vi "Graphs.vi"() -> ()   [LabVIEW 2020, in "Database Lib.lvlib"]
uses:
  Database Lib.lvlib
  <vilib>/Analysis/baseanly.llb/Mean (DBL).vi
  <vilib>/Analysis/NI_AALBase.lvlib
panel:
  out "XY Graph":cluster{"X":dbl, "Y":dbl}[](graph)
  out "Tab Control":enum32{"Histogram", "Length-Width", "Grading"}(tab)
  out "Diameter Histogram":cluster{"subarray":dbl[], dbl[]}(graph)
  in  "Menu":enum32{"Histogram", "Length-Width", "Grading"}(radio)
  in  "Close":bool
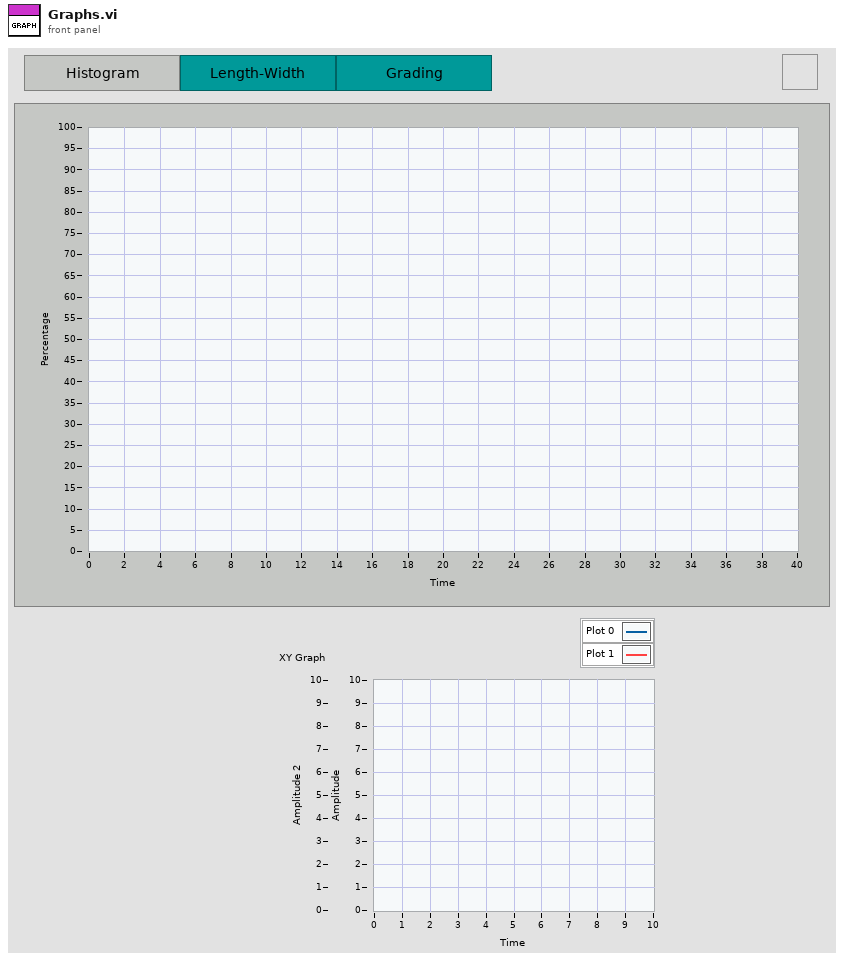
[diagram p1: front panel]
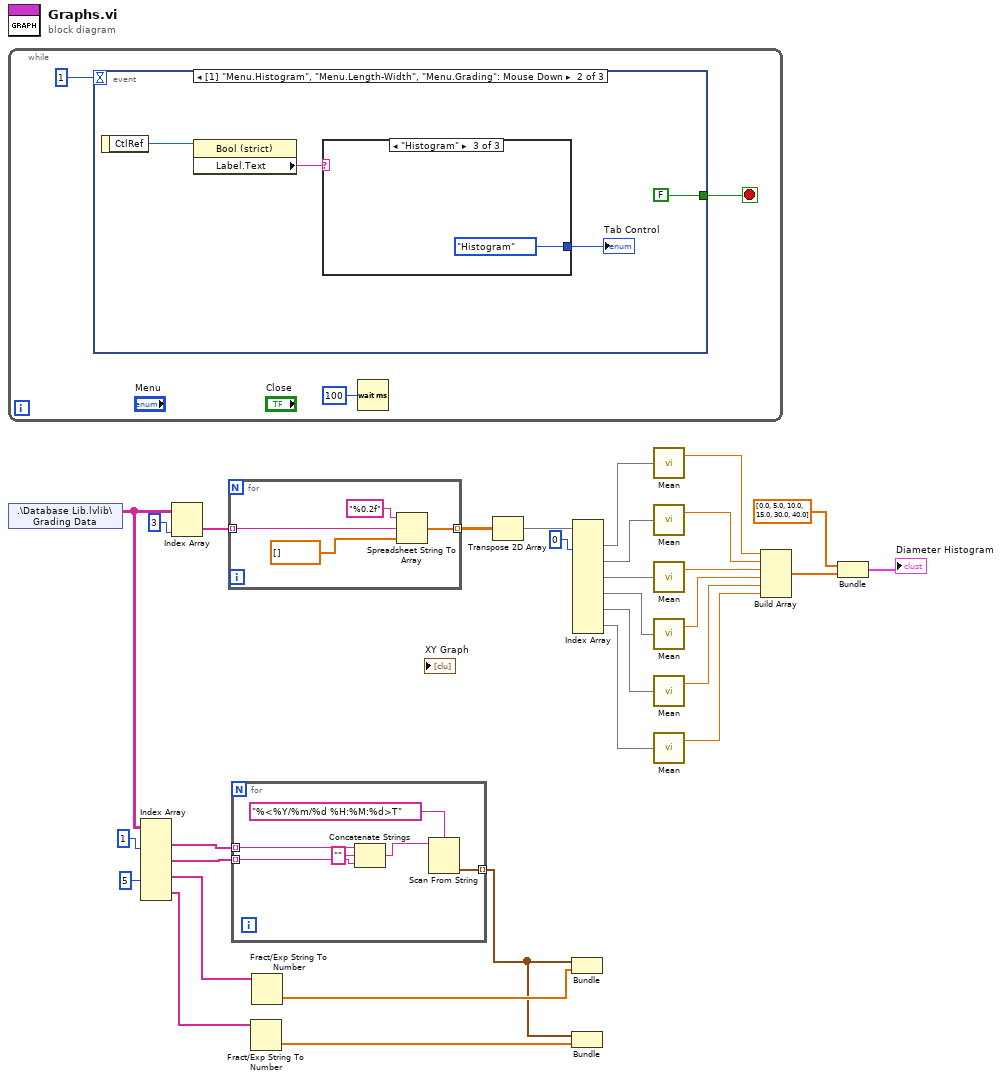
[diagram p0: block diagram]
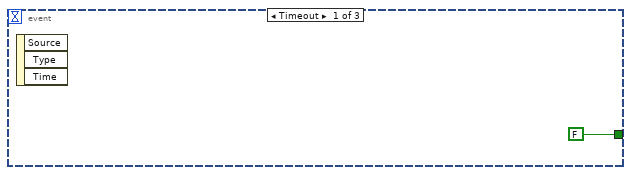
[diagram p2: hidden frame]
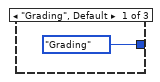
[diagram p3: hidden frame]
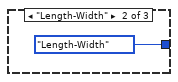
[diagram p4: hidden frame]
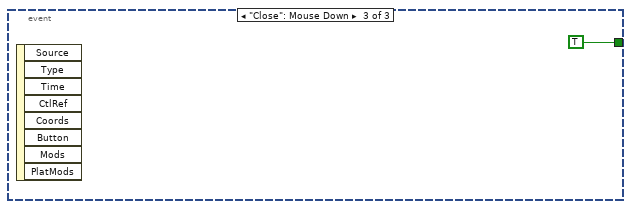
[diagram p5: hidden frame]
diagram:
  n1 = while {
    stop <- w32 stop-if-true
    n2 = event shown="[1] \"Menu.Histogram\", \"Menu.Length-Width\", \"Menu.Grading\": Mouse Down" {
      selector: _ -> [_ _ _]
      dyn-events: _ -> [_ _ _]
      timeout: 1 -> [_ _ _]
      tunnel: [FALSE FALSE TRUE] -> w32
      event Timeout {
        n3 = event-data() -> ()  [unwired: 1 in, 3 out]
      }
      event "Menu.Histogram", "Menu.Length-Width", "Menu.Grading": Mouse Down {
        n4 = event-data() -> ("CtlRef"=w37:refnum<vi>)  [unwired: 1 in]
        n5 = property class="Bool (strict)"(reference=w37) -> ("Label.Text"=w36:string)  [unwired: 1 in, 2 out]
        n6 = case shown="\"Histogram\"" w36 {
          tunnel: [enum32{"Histogram", "Length-Width", "Grading"}."Grading" ("Tab Control") enum32{"Histogram", "Length-Width", "Grading"}."Length-Width" ("Tab Control") enum32{"Histogram", "Length-Width", "Grading"}."Histogram" ("Tab Control")] -> w35
          frame "Grading", Default {
          }
          frame "Length-Width" {
          }
          frame "Histogram" {
          }
        }
        "Tab Control" <- w35
      }
      event "Close": Mouse Down {
        n7 = event-data() -> ()  [unwired: 1 in, 8 out]
      }
    }
    n8 = Wait (ms)(milliseconds to wait=u32 100) -> ()  [unwired: 1 out]
  }
  n9 = shared-variable ".\\Database Lib.lvlib\\Grading Data"() -> (w9:string[][])  [unwired: 1 in, 1 out]
  n10 = Index Array(array=w9, index (col) #1=1 ("disabled index (col)"), index (col) #3=5 ("index (col)")) -> (element #1=w8:string[], element #2=w7:string[], element #3=w5:string[], element #4=w4:string[])  [unwired: 6 in]
  n11 = Index Array(array=w9, index (col)=3 ("disabled index (col)")) -> (element=w29:string[])  [unwired: 1 in]
  n12 = for {
    tunnel: w29 -> [w46] mode=indexing
    tunnel: [w43] -> w28 mode=indexing
    n13 = Spreadsheet String To Array(format string="%0.2f", spreadsheet string=w46, array type (2D Dbl)=dbl[] []) -> (array=w43:dbl[])  [unwired: 1 in]
  }
  n14 = for {
    tunnel: w8 -> [w52] mode=indexing
    tunnel: w7 -> [w51] mode=indexing
    tunnel: [w47] -> w2 mode=indexing
    n15 = Concatenate Strings(w52, "" ("string"), w51) -> (w49:string)
    n16 = Scan From String(format string="%<%Y/%m/%d %H:%M:%d>T", input string=w49) -> (output 1=w47:timestamp)  [unwired: 3 in, 3 out]
  }
  n17 = Fract/Exp String To Number(string=w4) -> (number=w1:dbl[])  [unwired: 3 in, 1 out]
  n18 = Fract/Exp String To Number(string=w5) -> (number=w3:dbl[])  [unwired: 3 in, 1 out]
  n19 = Transpose 2D Array(2D array=w28) -> (transposed array=w27:dbl[][])
  n20 = Bundle(w2, w3) -> ()  [unwired: 1 in, 1 out]
  n21 = Bundle(w2, w1) -> ()  [unwired: 1 in, 1 out]
  n22 = Index Array(array=w27, index (col) #1=0 ("disabled index (col)")) -> (element #1=w25:dbl[], element #2=w24:dbl[], element #3=w23:dbl[], element #4=w22:dbl[], element #5=w21:dbl[], element #6=w20:dbl[])  [unwired: 11 in]
  n23 = call-poly <vilib>:"Mean.vi"("X"=w25) -> ("mean"=w19:dbl)  [unwired: 1 out]
  n24 = call-poly <vilib>:"Mean.vi"("X"=w24) -> ("mean"=w18:dbl)  [unwired: 1 out]
  n25 = call-poly <vilib>:"Mean.vi"("X"=w23) -> ("mean"=w17:dbl)  [unwired: 1 out]
  n26 = call-poly <vilib>:"Mean.vi"("X"=w22) -> ("mean"=w16:dbl)  [unwired: 1 out]
  n27 = call-poly <vilib>:"Mean.vi"("X"=w21) -> ("mean"=w15:dbl)  [unwired: 1 out]
  n28 = call-poly <vilib>:"Mean.vi"("X"=w20) -> ("mean"=w14:dbl)  [unwired: 1 out]
  n29 = Build Array(w19, w18, w17, w16, w15, w14) -> (w12:dbl[])
  n30 = Bundle("subarray"=dbl[] [0.0, 5.0, 10.0, 15.0, 30.0, 40.0], w12) -> (→"Diameter Histogram":cluster{"subarray":dbl[], dbl[]})  [unwired: 1 in]
